vi "CopyImage.vi"(8 "error in":errorcluster, 9 "Copy to Index":i32, 10 "Copy From Index":i32) -> (0 "error out":errorcluster, 4 "return":i32)   [LabVIEW 2015]
uses:
  [Global] Image.vi
  [Global] Image Overlay.vi
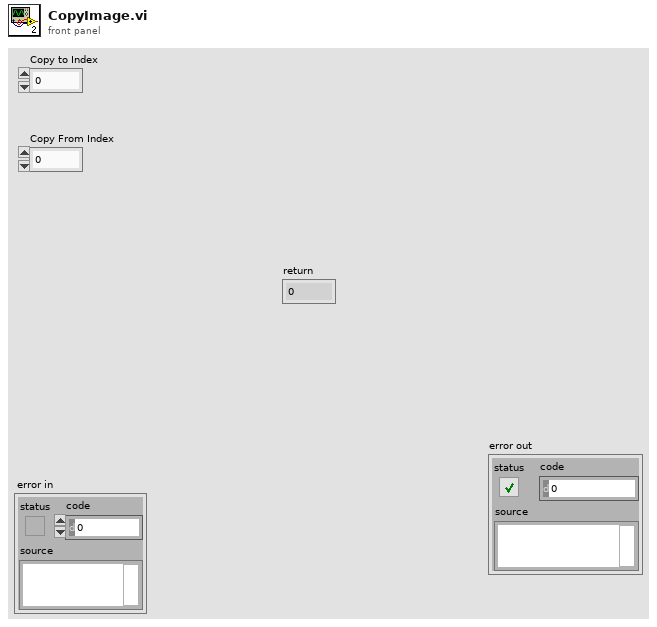
[diagram p1: front panel]
types:
  T1 = typedef "IMAQ Image.ctl" = refnum<image>
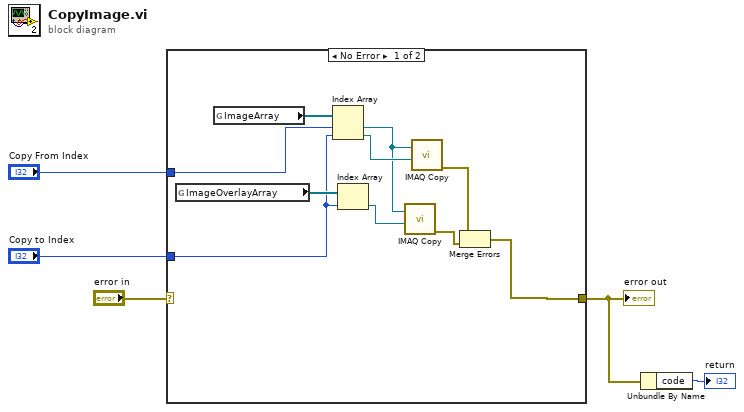
[diagram p0: block diagram]
diagram:
  n1 = case shown="No Error" "error in" {
    selector: "error in" -> [_ w16]
    tunnel: [w10 w16] -> w3
    tunnel: "Copy From Index" -> [w11 _]
    tunnel: "Copy to Index" -> [w7 _]
    frame No Error {
      n2 = global read "[Global] Image Overlay.vi" "ImageOverlayArray"() -> (w12:T1[])
      n3 = global read "[Global] Image.vi" "ImageArray"() -> (w15:T1[])
      n4 = Index Array(array=w15, index #1=w11, index #2=w7) -> (element #1=w8:T1, element #2=w14:T1)
      n5 = Index Array(array=w12, index=w7) -> (element=w6:T1)
      n6 = call "IMAQ Copy"("Image Dst"=w6, "Image Src"=w8) -> ("error out"=w9:errorcluster)  [unwired: 4 in, 1 out]
      n7 = call "IMAQ Copy"("Image Dst"=w14, "Image Src"=w8) -> ("error out"=w13:errorcluster)  [unwired: 4 in, 1 out]
      n8 = Merge Errors(w13, w9) -> (w10:errorcluster)
    }
    frame Error {
    }
  }
  "error out" <- w3
  n9 = Unbundle By Name(w3) -> ("code"=→"return":i32)
